vi "GetSecurityMode.vi"(0 "reference in":refnum<class "Security.lvclass">, 5 "Error In":errorcluster) -> (14 "reference out":refnum<class "Security.lvclass">, 16 "Security Mode":T1, 19 "Error Out":errorcluster)   [LabVIEW 2024, in "Security.lvclass"]
uses:
  Security.lvclass
  Security.lvclass/Security.ctl
  Systems/SecuritySystem_class/Security Mode.ctl
  Systems/SecuritySystem_class/SecuritySystem.lvclass
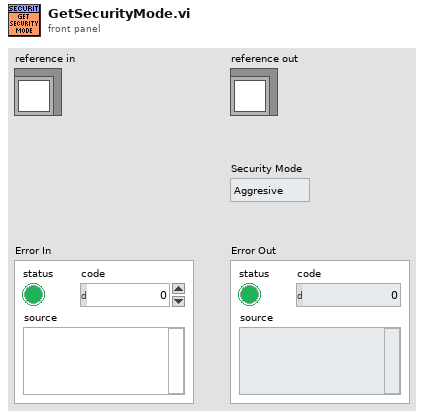
[diagram p1: front panel]
types:
  T1 = typedef "SecuritySystem.lvclass/Security Mode.ctl" = enum16{"Aggresive", "Defensive", "Balanced"}
  T2 = typedef "Security.lvclass/ObjectAttributes.ctl" = cluster{"State":bool, "Security Mode":T1}
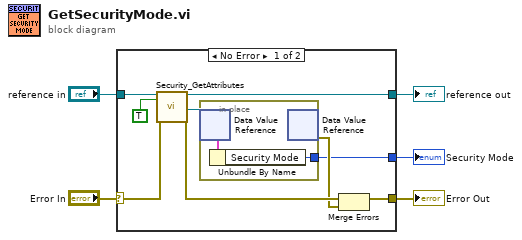
[diagram p0: block diagram]
diagram:
  n1 = case shown="No Error" "Error In" {
    selector: "Error In" -> [w14 w18]
    tunnel: [w12 w18] -> w4
    tunnel: [w9 w17] -> w2
    tunnel: "reference in" -> [w10 w17]
    tunnel: [w6 _] -> w1
    frame No Error {
      n2 = call "Security_GetAttributes.vi"("reference in"=w10, "OnlyGetDvrReference(False)"=TRUE, "Error In"=w14) -> ("reference out"=w9:refnum<class "Security.lvclass">, "DataRef"=w8:refnum<data-value>, "Error Out"=w13:errorcluster)  [unwired: 13 in, 1 out]
      n3 = in-place {
        in-place-border: [w16] -> w6
        n4 = in-place-dvr #1(w8) -> (w15:T2)  [unwired: 1 out]
        n5 = Unbundle By Name(w15) -> ("Security Mode"=w16:T1)
        n6 = in-place-dvr #1() -> (w11:errorcluster)  [unwired: 1 in, 1 out]
      }
      n7 = Merge Errors(w13, w11) -> (w12:errorcluster)
    }
    frame Error {
    }
  }
  "Error Out" <- w4
  "reference out" <- w2
  "Security Mode" <- w1
